vi "table color.vi"(11 "Line 2":refnum<vi>) -> ()   [LabVIEW 2015]
uses:
  <vilib>/Utility/miscctls.llb/LVRowAndColumnTypeDef.ctl
panel:
  in  "Line 1":string[][](table)
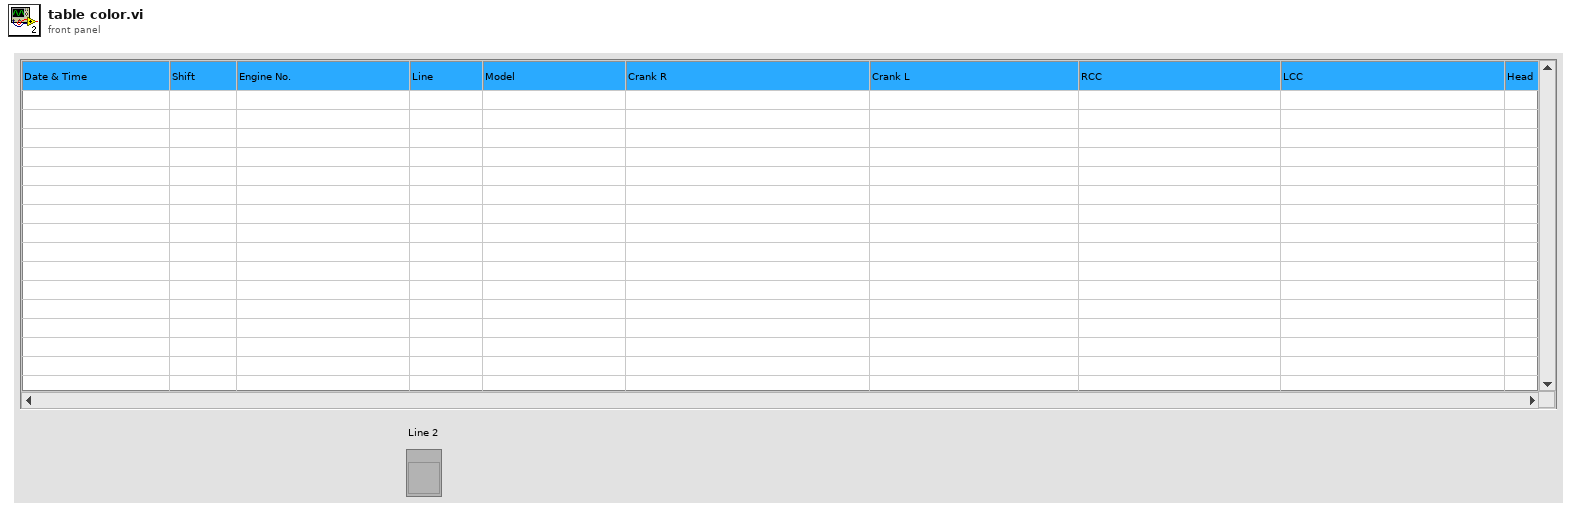
[diagram p1: front panel]
types:
  T1 = typedef "LVRowAndColumnTypeDef.ctl" = cluster{"Row":i32, "Column":i32}
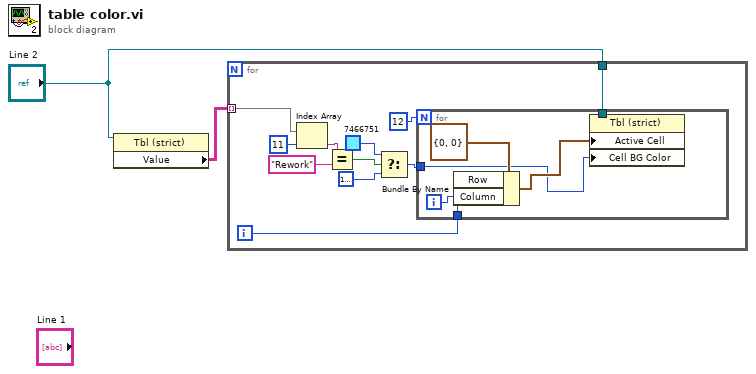
[diagram p0: block diagram]
diagram:
  n1 = property class="Tbl (strict)"(reference="Line 2") -> ("Value"=w2:string[][])  [unwired: 1 in, 2 out]
  n2 = for {
    tunnel: w2 -> [w13] mode=indexing
    tunnel: "Line 2" -> [w3]
    i -> [w11]
    n3 = Index Array(array=w13, index=11) -> (element=w10:string)
    n4 = Equal?(x=w10, y="Rework") -> (x = y?=w7:bool)
    n5 = Select(t=u32 7466751, s=w7, f=u32 16777225) -> (s? t:f=w4:u32)
    n6 = for {
      N: 12 -> [_]
      tunnel: w11 -> [w18]
      tunnel: w4 -> [w14]
      tunnel: w3 -> [w16]
      i -> [w17]
      n7 = Bundle By Name(cluster=T1 {"Row"=0, "Column"=0} ("Active Cell:Active Cell"), "Row"=w18, "Column"=w17) -> (w15:T1)
      n8 = property class="Tbl (strict)"(reference=w16, "Active Cell"=w15, "Cell BG Color"=w14) -> ()  [unwired: 1 in, 2 out]
    }
  }
